vi "Execute.vi"(6 "Error":errorcluster, 7 "ConcreteMessage":refnum<class "ConcreteMessage.lvclass">, 11 "Actor":refnum<class "Actor.lvclass">) -> (3 "Actor":refnum<class "Actor.lvclass">, 4 "Error":errorcluster, 5 "ConcreteMessage":refnum<class "ConcreteMessage.lvclass">)   [LabVIEW 2020, in "_Template.lvlib" / "MessageTemplate.lvlib" / "{{Name}}.lvlib" / "ConcreteMessage.lvclass"]
uses:
  ConcreteMessage.lvclass
  jettl/jettl/Actor/Actor.lvclass
  Message/Message.lvclass
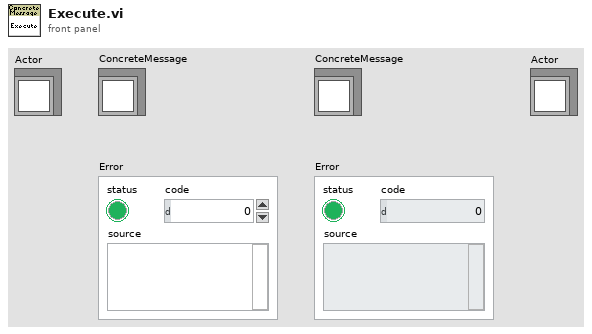
[diagram p1: front panel]
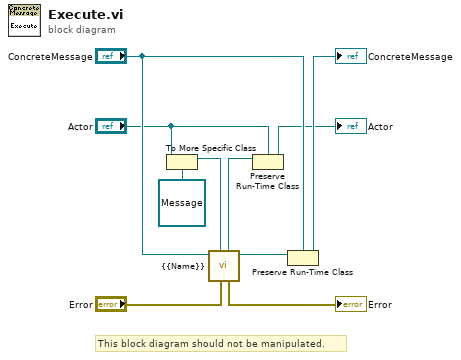
[diagram p0: block diagram]
diagram:
  # "This block diagram should not be manipulated."
  n1 = To More Specific Class(target class=refnum<class "Message.lvclass"> refnum ("_Template.lvlib:Templates.lvlib:TEMPLATE jettl Msg.lvlib:TEMPLATE jettl Msg.lvclass"), reference="Actor") -> (specific class reference=w7:refnum<class "Message.lvclass">)  [unwired: 1 in, 1 out]
  n2 = call-dynamic "{{Name}}.vi"("Error"="Error", "Message"=w7, "ConcreteMessage"="ConcreteMessage") -> ("ConcreteMessage"=w4:refnum<class "ConcreteMessage.lvclass">, "Error"=→"Error":errorcluster, "Message"=w6:refnum<class "Message.lvclass">)  [unwired: 6 in]
  n3 = Preserve Run-Time Class(object in=w6, 2:"Actor") -> (object out=→"Actor":refnum<class "Actor.lvclass">)  [unwired: 1 in, 1 out]
  n4 = Preserve Run-Time Class(object in=w4, 2:"ConcreteMessage") -> (object out=→"ConcreteMessage":refnum<class "ConcreteMessage.lvclass">)  [unwired: 1 in, 1 out]
